vi "HFRR ADV v07.vi"() -> ()   [LabVIEW 2025] (continued)
                n2727 = local read "export"() -> (w3522:string)
                n2728 = call <vilib>:"Write Characters To File.vi"("append to file? (new file:F)"=FALSE, "character string"=w3522, "file path (dialog if empty)"=w3527) -> ()  [unwired: 2 in, 1 out]
              }
            }
          }
          frame Enabled {
          }
        }
        n2729 = case shown="True" "OK Button 17" {
          frame False {
          }
          frame True {
            (unwired) 0  # existing file
            w3780 = "Choose a datalog file to open"  # prompt
            n2730 = local write "OK Button 17"(FALSE ("OK Button 17")) -> ()
            n2731 = local read "String"() -> (w3775:string)
            n2732 = String To Path(string=w3775) -> (path=w3776:path)
            n2733 = File Dialog(6:"*.duf" ("pattern"), 7:w3780, 11:w3776) -> (0:w3767:errorcluster, 3:w3786:path)  [unwired: 4 in, 2 out]
            n2734 = Unbundle(w3767) -> ()  [unwired: 3 out]
            n2735 = Open/Create/Replace File "Open File"(file path (use dialog)=w3786) -> (refnum out=w3778:refnum<file>)  [unwired: 5 in, 2 out]
            n2736 = Strip Path(path=w3786) -> (name=w3784:string)  [unwired: 1 out]
            n2737 = Path To String(path=w3786) -> (string=w3769:string)
            n2738 = local write "String 29"(w3769) -> ()
            n2739 = while {
              tunnel: w3778 -> [w3790]
              i -> [w3787]
              stop <- w3788 continue-if-true
              (unwired) TRUE ("line mode (F)")
              n2740 = Read from Text File "Read File"(file (use dialog)=w3790) -> (text=w3789:string)  [unwired: 3 in, 3 out]
              n2741 = local write "Numeric 16"(w3787) -> ()
              n2742 = String Length(string=w3789) -> (length=w3792:i32)
              n2743 = Greater?(x=w3792, y=1) -> (0:w3788:bool)
            }
            n2744 = Search and Replace String(input string=w3769, search string=".duf", replace string=".dgf" ("replace string (\"\")")) -> (result string=→"String Indicator 4":string)  [unwired: 5 in, 3 out]
            n2745 = Match Pattern(string=w3784, regular expression=".dwm") -> (before substring=w3768:string)  [unwired: 1 in, 3 out]
            "String Indicator" <- w3768
            n2746 = Match Pattern(string=w3769, regular expression=".dwm" ("substring (\"\")")) -> (before substring=w3770:string)  [unwired: 1 in, 3 out]
            "String Indicator 3" <- w3770
            n2747 = local write "TITTLE 2"(w3768) -> ()
            n2748 = String To Path(string=w3770) -> (path=w3777:path)
            "path" <- w3777
            n2749 = call <vilib>:"Read Characters From File.vi"("file path (dialog if empty)"=w3777, "start of read offset (chars.:0)"=60 ("start of read offset (chars.: 0)")) -> ("character string"=→"String Indicator 2":string)  [unwired: 4 in, 3 out]
          }
        }
        n2750 = case shown="True" "Print 2" {
          frame False {
          }
          frame True {
            n2751 = flat-sequence {
              frame #0 {
                n2752 = local read "s.NO"() -> (→"s.NO 2":string)
                n2753 = Wait (ms)(milliseconds to wait=u32 20) -> ()  [unwired: 1 out]
                n2754 = local read "Sample ID  4"() -> (→"Sample ID  7":string)
                n2755 = local read "Sample ID  3"() -> (→"Sample ID  6":string)
                n2756 = local read "Sample ID"() -> (→"Sample ID  2":string)
                n2757 = local read "Tested by"() -> (→"Tested by 2":string)
                n2758 = local read "Test Date"() -> (→"Test Date 2":string)
                n2759 = local read "Humidity after test 3"() -> (→"Humidity after test 4":dbl)
                n2760 = local read "Ref A Test Date :"() -> (→"TITTLE 4":string)
                n2761 = local read "Temperature before test 3"() -> (→"Temperature after test 5":dbl)
                n2762 = local read "Temperature before test 3"() -> (w3588:dbl)
                n2763 = local read "Temperature after test 3"() -> (→"Temperature after test 4":dbl)
                n2764 = local read "Humidity before test 3"() -> (→"Humidity before test 4":dbl)
                n2765 = local write "Temperature before test 3"(w3588) -> ()
                n2766 = local read "image data"() -> (w3579:T13)
                n2767 = String To Path(string="C:\\LAB-IQ\\im\\Temp_resized.jpg") -> (path=w3580:path)
                "path 2" <- w3580
                n2768 = call <vilib>:"Write JPEG File.vi"("image data"=w3579, "path to JPEG file"=w3580) -> ()  [unwired: 8 in, 2 out]
                "Ref A Test Date :" <- "Ref A Test Date :"
                "Ref B Test Date :" <- "Ref B Test Date :"
                "Ref B Scar Value :" <- "Ref B Scar Value :"
                "Ref A Scar Value :" <- "Ref A Scar Value :"
              }
              frame #1 {
                (unwired) HTML_Report_Image_Alignment."MIDDLE" ("alignment (default)")
                w3616 = u16 0 items=["portrait", "landscape"] ("orientation (portrait)")
                (unwired) HTML_Report_Image_Alignment."ABSMIDDLE" ("alignment (default)")
                (unwired) "TESTED BY : "
                (unwired) "TESTED DATE :"
                (unwired) "SAMPLE ID : "
                (unwired) "SAMPLE DESIGN : "
                w3649 = "\r"
                # "add image"
                n2769 = Wait (ms)(milliseconds to wait=u32 20) -> ()  [unwired: 1 out]
                n2770 = local read "Sample ID  2"() -> (w3642:string)
                n2771 = local read "Wear Scar X"() -> (w3614:dbl)
                "Length ( microns ) 2" <- w3614
                n2772 = local read "Wear Scar Y"() -> (w3613:dbl)
                "Wear Scar Y ( microns ) :" <- w3613
                n2773 = local read "Test Date 2"() -> (w3643:string)
                n2774 = local read "Tested by 2"() -> (w3644:string)
                n2775 = local read "String 46"() -> (w3640:string)
                n2776 = local read "String 47"() -> (w3645:string)
                n2777 = local read "String 48"() -> (w3646:string)
                n2778 = local read "String 49"() -> (w3647:string)
                n2779 = local read "String 10"() -> (w3600:string)
                n2780 = local read "s.NO 2"() -> (w3641:string)
                n2781 = Add(x=w3614, y=w3613) -> (x+y=w3612:dbl)
                n2782 = call <vilib>:"New Report.vi"("report type"=enum16{"Standard Report", "HTML"}."HTML") -> ("report out"=w3620:refnum<class "NI_report.lvclass">, "error out"=w3618:errorcluster)  [unwired: 13 in]
                n2783 = Concatenate Strings(w3649, w3640, w3641, w3649, w3646, w3642, w3649, w3645, w3643, w3649, w3647, w3644, w3649) -> (→"test by 2":string)
                n2784 = Concatenate Strings("C:\\LAB-IQ\\Data\\" ("string"), w3600, ".jpg" ("string")) -> ()  [unwired: 1 out]
                n2785 = Divide(x=w3612, y=2.0) -> (x/y=→"Mean Wear ( microns) :":dbl)
                n2786 = call-dynamic "Set Report Orientation.vi"("report in"=w3620, "orientation (portrait)"=w3616, "error in (no error)"=w3618) -> ("report out"=w3619:refnum<class "NI_report.lvclass">, "error out"=w3617:errorcluster)  [unwired: 11 in]
                n2787 = for {
                  N: 5 -> [_]
                  tunnel: w3619 -> [w3670]
                  tunnel: [w3669] -> w3598
                  tunnel: w3617 -> [w3668]
                  tunnel: [w3667] -> w3597
                  n2788 = call-dynamic "Set Report Tab Width.vi"("report in"=w3670, "error in (no error)"=w3668) -> ("report out"=w3669:refnum<class "NI_report.lvclass">, "error out"=w3667:errorcluster)  [unwired: 12 in]
                }
                n2789 = local read "TITTLE"() -> (w3615:string)
                n2790 = call-dynamic "Set Report Header Text.vi"("report in"=w3598, "center header text"=w3615, "error in (no error)"=w3597) -> ("report out"=w3636:refnum<class "NI_report.lvclass">, "error out"=w3635:errorcluster)  [unwired: 11 in]
                n2791 = for {
                  N: 1 -> [_]
                  tunnel: [w3674] -> w3622
                  tunnel: [w3673] -> w3621
                  tunnel: w3636 -> [w3672]
                  tunnel: w3635 -> [w3671]
                  n2792 = call-dynamic "New Report Line.vi"("report in"=w3672, "error in (no error)"=w3671) -> ("report out"=w3674:refnum<class "NI_report.lvclass">, "error out"=w3673:errorcluster)  [unwired: 12 in]
                }
                n2793 = for {
                  N: 2 -> [_]
                  tunnel: [w3666] -> w3628
                  tunnel: [w3665] -> w3627
                  tunnel: w3622 -> [w3664]
                  tunnel: w3621 -> [w3663]
                  n2794 = call-dynamic "New Report Line.vi"("report in"=w3664, "error in (no error)"=w3663) -> ("report out"=w3666:refnum<class "NI_report.lvclass">, "error out"=w3665:errorcluster)  [unwired: 12 in]
                }
                n2795 = for {
                  N: 25 -> [_]
                  tunnel: w3628 -> [w3662]
                  tunnel: w3627 -> [w3660]
                  tunnel: [w3661] -> w3631
                  tunnel: [w3659] -> w3630
                  n2796 = call-dynamic "Set Report Tab Width.vi"("report in"=w3662, "error in (no error)"=w3660) -> ("report out"=w3661:refnum<class "NI_report.lvclass">, "error out"=w3659:errorcluster)  [unwired: 12 in]
                }
                n2797 = control-ref of="Tab Control 9"() -> (w3626:refnum<vi>)
                n2798 = call-dynamic "Append Control Image to Report.vi"("report in"=w3631, "alignment (default)"=HTML_Report_Image_Alignment."ABSMIDDLE", "ctrl reference"=w3626, "error in (no error)"=w3630) -> ("report out"=w3625:refnum<class "NI_report.lvclass">, "error out"=w3624:errorcluster)  [unwired: 8 in, 2 out]
                n2799 = for {
                  N: 3 -> [_]
                  tunnel: [w3658] -> w3609
                  tunnel: [w3657] -> w3608
                  tunnel: w3625 -> [w3656]
                  tunnel: w3624 -> [w3655]
                  n2800 = call-dynamic "New Report Line.vi"("report in"=w3656, "error in (no error)"=w3655) -> ("report out"=w3658:refnum<class "NI_report.lvclass">, "error out"=w3657:errorcluster)  [unwired: 12 in]
                }
                n2801 = for {
                  N: 100 -> [_]
                  tunnel: w3609 -> [w3654]
                  tunnel: w3608 -> [w3652]
                  tunnel: [w3653] -> w3605
                  tunnel: [w3651] -> w3603
                  n2802 = call-dynamic "Set Report Tab Width.vi"("report in"=w3654, "error in (no error)"=w3652) -> ("report out"=w3653:refnum<class "NI_report.lvclass">, "error out"=w3651:errorcluster)  [unwired: 12 in]
                }
                n2803 = String To Path(string="C:\\LAB-IQ\\im\\Temp_resized.jpg") -> (path=w3595:path)
                n2804 = call-poly <vilib>:"Append Image to Report.vi"("report in"=w3605, "path or URL of image"=w3595, "error in (no error)"=w3603) -> ("report out"=w3604:refnum<class "NI_report.lvclass">, "error out"=w3602:errorcluster)  [unwired: 9 in, 2 out]
                n2805 = call-poly <vilib>:"Open HTML Report in Browser.vi"("report in"=w3604, "error in (no error)"=w3602) -> ("report out"=w3639:refnum<class "NI_report.lvclass">, "error out"=w3638:errorcluster)  [unwired: 11 in, 1 out]
                n2806 = call-dynamic "Dispose Report.vi"("report in"=w3639, "error in (no error)"=w3638) -> ()  [unwired: 13 in, 1 out]
              }
              frame #2 {
              }
              frame #3 {
                n2807 = local write "Print 2"(FALSE ("Print")) -> ()
                n2808 = disable-structure shown="Disabled" {
                  frame Disabled {
                    n2809 = local read "String 10"() -> (w3679:string)
                    n2810 = Concatenate Strings("C:\\LAB-IQ-NXT\\Data\\" ("string"), w3679, ".jpg" ("string")) -> (w3677:string)
                    n2811 = String To Path(string=w3677) -> (path=w3676:path)
                    n2812 = Delete(path (use dialog)=w3676) -> ()  [unwired: 4 in, 3 out]
                  }
                  frame Enabled {
                  }
                }
              }
            }
          }
        }
        n2813 = case shown="True" w3466 {
          frame False {
          }
          frame True {
            n2814 = flat-sequence {
              frame #0 {
              }
              frame #1 {
                n2815 = Wait (ms)(milliseconds to wait=u32 100) -> ()  [unwired: 1 out]
              }
              frame #2 {
                n2816 = local write "OK Button 16"(FALSE ("Print 3")) -> ()
              }
            }
          }
        }
        n2817 = case shown="True" "Print" {
          tunnel: w3471 -> [_ w3763]
          frame False {
          }
          frame True {
            (unwired) i16 6 ("width (-)")
            (unwired) "TESTED BY : "
            (unwired) "TESTED DATE :"
            (unwired) "SAMPLE ID : "
            (unwired) "SAMPLE DESIGN : "
            w3721 = "\r"
            w3738 = "\r"
            # "add image"
            n2818 = local read "Sample ID"() -> (w3711:string)
            n2819 = local read "Tested by"() -> (w3714:string)
            n2820 = local read "String 45"() -> (w3681:string)
            n2821 = local read "Test Date"() -> (w3712:string)
            n2822 = local read "String 39"() -> (w3684:string)
            n2823 = local read "String 38"() -> (w3687:string)
            n2824 = local read "String 37"() -> (w3694:string)
            n2825 = local read "String 36"() -> (w3691:string)
            n2826 = local read "String 35"() -> (w3696:string)
            n2827 = local read "String 34"() -> (w3701:string)
            n2828 = local read "String 31"() -> (w3715:string)
            n2829 = local read "String 32"() -> (w3716:string)
            n2830 = local read "String 33"() -> (w3717:string)
            n2831 = local write "Print"(FALSE ("Print FF")) -> ()
            n2832 = local read "S 39"() -> (w3699:string)
            n2833 = local read "S 38"() -> (w3706:string)
            n2834 = local read "Temperature before test 2"() -> (w3737:dbl)
            n2835 = local read "Temperature after test 2"() -> (w3727:dbl)
            n2836 = local read "Humidity before test 2"() -> (w3752:dbl)
            n2837 = local read "Humidity after test 2"() -> (w3736:dbl)
            n2838 = local read "MWSD 2"() -> (w3741:dbl)
            n2839 = local read "WS1.4 2"() -> (w3719:dbl)
            n2840 = Concatenate Strings("8)" ("string"), w3684) -> (w3685:string)
            n2841 = Concatenate Strings("7)" ("string"), w3687) -> (w3688:string)
            n2842 = Concatenate Strings("6)" ("string"), w3691) -> (w3690:string)
            n2843 = Concatenate Strings("5)" ("string"), w3694) -> (w3693:string)
            n2844 = Concatenate Strings("4)" ("string"), w3696) -> (w3697:string)
            n2845 = Concatenate Strings("3)" ("string"), w3699) -> (w3700:string)
            n2846 = Concatenate Strings("2)" ("string"), w3701) -> (w3702:string)
            n2847 = Concatenate Strings("1)" ("string"), w3706) -> (w3705:string)
            n2848 = local read "HCF 2"() -> (w3723:dbl)
            n2849 = local read "AVP 2"() -> (w3740:dbl)
            n2850 = local read "s.NO"() -> (w3682:string)
            n2851 = call <vilib>:"New Report.vi"("report type"=enum16{"Standard Report", "HTML"}."Standard Report") -> ("report out"=w3761:refnum<class "NI_report.lvclass">, "error out"=w3760:errorcluster)  [unwired: 13 in]
            n2852 = local read "TITTLE"() -> (w3713:string)
            n2853 = Concatenate Strings(w3738, w3681, w3682, w3738, w3716, w3711, w3738, w3715, w3712, w3738, w3717, w3714, w3738) -> (w3731:string)
            "test by" <- w3731
            n2854 = Number To Fractional String(number=w3719, precision (6)=i16 2) -> (F-format string=w3718:string)  [unwired: 2 in]
            n2855 = Number To Fractional String(number=w3723, width (-)=i16 6, precision (6)=i16 2) -> (F-format string=w3722:string)  [unwired: 1 in]
            n2856 = Number To Fractional String(number=w3727, width (-)=i16 6, precision (6)=i16 2) -> (F-format string=w3728:string)  [unwired: 1 in]
            n2857 = Number To Fractional String(number=w3740, width (-)=i16 6, precision (6)=i16 2) -> (F-format string=w3742:string)  [unwired: 1 in]
            n2858 = Number To Fractional String(number=w3741, width (-)=i16 6, precision (6)=i16 2) -> (F-format string=w3743:string)  [unwired: 1 in]
            n2859 = Number To Fractional String(number=w3736, width (-)=i16 6, precision (6)=i16 2) -> (F-format string=w3739:string)  [unwired: 1 in]
            n2860 = Number To Fractional String(number=w3737, width (-)=i16 6, precision (6)=i16 2) -> (F-format string=w3726:string)  [unwired: 1 in]
            n2861 = Number To Fractional String(number=w3752, width (-)=i16 6, precision (6)=i16 2) -> (F-format string=w3757:string)  [unwired: 1 in]
            n2862 = call-dynamic "Set Report Header Text.vi"("report in"=w3761, "center header text"=w3713, "error in (no error)"=w3760) -> ("report out"=w3732:refnum<class "NI_report.lvclass">, "error out"=w3733:errorcluster)  [unwired: 11 in]
            n2863 = Concatenate Strings(w3721, w3705, w3757, w3721, w3702, w3726, w3721, w3700, w3739, w3721, w3697, w3728, w3721, w3693, w3743, w3721, w3690, w3742, w3721, w3688, w3722, w3721, w3685, w3718) -> (w3709:string)
            "export 2" <- w3709
            n2864 = call-poly <vilib>:"Append Report Text.vi"("report in"=w3732, "text"=w3731, "error in (no error)"=w3733) -> ("report out"=w3735:refnum<class "NI_report.lvclass">, "error out"=w3734:errorcluster)  [unwired: 9 in, 2 out]
            n2865 = local read "test by"() -> (w3708:string)
            n2866 = local read "TITTLE"() -> (w3710:string)
            n2867 = call-poly <vilib>:"Append Report Text.vi"("report in"=w3735, "error in (no error)"=w3734) -> ("report out"=w3756:refnum<class "NI_report.lvclass">, "error out"=w3754:errorcluster)  [unwired: 10 in, 2 out]
            n2868 = Concatenate Strings(w3710, w3709, w3708) -> (→"output":string)
            n2869 = call-poly <vilib>:"Append Report Text.vi"("report in"=w3756, "text"=w3709, "error in (no error)"=w3754) -> ("report out"=w3755:refnum<class "NI_report.lvclass">, "error out"=w3753:errorcluster)  [unwired: 9 in, 2 out]
            n2870 = call-dynamic "Print Report.vi"("report in"=w3755, "printer name (default)"=w3763, "error in (no error)"=w3753) -> ("report out"=w3765:refnum<class "NI_report.lvclass">, "error out"=w3766:errorcluster)  [unwired: 11 in]
            n2871 = call-dynamic "Dispose Report.vi"("report in"=w3765, "error in (no error)"=w3766) -> ()  [unwired: 13 in, 1 out]
          }
        }
      }
    }
    n2872 = case shown="True" "Prog Uno" {
      frame False {
      }
      frame True {
        n2873 = stacked-sequence {
          frame #0 {
            n2874 = Delete(path (use dialog)=path "C:/LAB-IQ-NXT/UNOCOMPILE.bat" ("working directory")) -> ()  [unwired: 4 in, 3 out]
          }
          frame #1 {
            n2875 = local read "Com Port 1"() -> (w2226:refnum<visa-resource-name>)
            n2876 = Concatenate Strings("cmd.exe /c \"mode " ("command line"), w2226, ":1200,n,8,1\"\n" ("command line")) -> (w2231:string)
            n2877 = Concatenate Strings(w2231, "CD\\\nCD WinDucom\navrdude -C avrdude.conf -v -patmega328p -carduino -P" ("command line"), w2226, " -b115200 -D -Uflash:w:UNO_V20.hex:i\n" ("command line"), "\r") -> (w2233:string)
            "STR" <- w2233
            n2878 = call <vilib>:"Write Characters To File.vi"("append to file? (new file:F)"=FALSE, "character string"=w2233, "file path (dialog if empty)"=path "C:/LAB-IQ/UNOCOMPILE.bat" ("working directory")) -> ()  [unwired: 2 in, 1 out]
          }
          frame #2 {
            n2879 = disable-structure shown="Disabled" {
              frame Disabled {
                w2237 = "cmd.exe  /c \"C:\\LAB-IQ-NXT\\UNOCOMPILE.bat\"" ("string")
                n2880 = local write "Prog Uno"(FALSE ("run minimized? (F)")) -> ()
                n2881 = call <vilib>:"System Exec.vi"("expected output size  (4096)"=u32 65535, "run minimized? (F)"=FALSE, "wait until completion? (T)"=TRUE ("run minimized? (F)"), "working directory"=path "C:/LAB-IQ-NXT", "standard input"=w2237, "command line"=w2237) -> ("error out"=w2236:errorcluster, "standard output"=→"String 42":string)  [unwired: 2 in, 2 out]
                "error out 3" <- w2236
                n2882 = flat-sequence {
                  tunnel: w2236 -> [_]
                  frame #0 {
                  }
                }
              }
              frame Enabled {
              }
            }
          }
        }
      }
    }
    n2883 = case shown="True" "Prog Due" {
      frame False {
      }
      frame True {
        n2884 = stacked-sequence {
          frame #0 {
            n2885 = Delete(path (use dialog)=path "C:/LAB-IQ/DUECOMPILE.bat" ("working directory")) -> ()  [unwired: 4 in, 3 out]
          }
          frame #1 {
            n2886 = disable-structure shown="Disabled" {
              frame Disabled {
                n2887 = local read "visa due"() -> (w2208:string)
                n2888 = Concatenate Strings("cmd.exe /c \"mode " ("command line"), w2208, ":1200,n,8,1\"\n" ("command line")) -> (w2213:string)
                n2889 = Concatenate Strings(w2213, "CD\\\nCD WinDucom\nTIMEOUT 1\n bossac.exe -i -d --port=" ("command line"), w2208, " -U false -e -w -v -b DUE.bin -R\n" ("command line"), "\r") -> (w2215:string)
                "concatenated string 2" <- w2215
                n2890 = call <vilib>:"Write Characters To File.vi"("append to file? (new file:F)"=FALSE, "character string"=w2215, "file path (dialog if empty)"=path "C:/LAB-IQ-NXT/DUECOMPILE.bat" ("working directory")) -> ()  [unwired: 2 in, 1 out]
              }
              frame Enabled {
              }
            }
          }
          frame #2 {
            # "C:\\LAB-IQ-NXT\\DUECOMPILE.bat"
            n2891 = local write "Prog Due"(FALSE ("Prog Due")) -> ()
            n2892 = disable-structure shown="Disabled" {
              frame Disabled {
                w2220 = "cmd.exe  /c \"C:\\LAB-IQ-NXT\\DUECOMPILE.bat\"" ("string")
                n2893 = call <vilib>:"System Exec.vi"("expected output size  (4096)"=u32 65535, "run minimized? (F)"=FALSE, "wait until completion? (T)"=TRUE ("run minimized? (F)"), "working directory"=path "C:/LAB-IQ-NXT", "standard input"=w2220, "command line"=w2220) -> ("error out"=w2219:errorcluster, "standard output"=→"String 44":string)  [unwired: 2 in, 2 out]
                "error out 4" <- w2219
                n2894 = flat-sequence {
                  tunnel: w2219 -> [_]
                  frame #0 {
                  }
                }
              }
              frame Enabled {
              }
            }
          }
        }
      }
    }
    n2895 = property on="SetTemp" class="DigNum (strict)"("Disabled"=w1630) -> ()  [unwired: 2 in, 2 out]
    n2896 = Multiply(x=w1620, y=w1622) -> (x*y=w1621:dbl)
    n2897 = local read "MWSD"() -> (w1619:dbl)
    n2898 = Add(x=w1621, y=w1619) -> (x+y=→"WS1.4":dbl)
    n2899 = Wait (ms)(milliseconds to wait=u32 50) -> ()  [unwired: 1 out]
    n2900 = Wait (ms)(milliseconds to wait=u32 50) -> ()  [unwired: 1 out]
    n2901 = local read "Quit"() -> (w1618:bool)
  }
  n2902 = while {
    tunnel: [w3838] -> w46
    shift-right: [w3831] -> _
    shift-left: 0.0 -> [w3834]
    shift-right: [w3830] -> _
    shift-left: 0.0 -> [w3833]
    shift-right: [w3829] -> _
    shift-left: 400.0 ("vc_cmd") -> [w3832]
    stop <- w3838 stop-if-true
    # "PID LOGIC"
    n2903 = local read "RUN"() -> (w3836:bool)
    n2904 = local read "Auto Start Test"() -> (w3835:bool)
    n2905 = local read "START TEMP"() -> (w3827:bool)
    n2906 = Or(x=w3836, y=w3835) -> (x .or. y?=w3837:bool)
    n2907 = And(x=w3837, y=w3827) -> (x .and. y?=w3828:bool)
    n2908 = case shown="True" w3828 {
      tunnel: [400.0 ("out_vc_cmd") w3858] -> w3829
      tunnel: [w3841 w3860] -> w3830
      tunnel: [w3841 w3859] -> w3831
      tunnel: w3834 -> [_ w3848]
      tunnel: w3833 -> [_ w3847]
      tunnel: w3832 -> [_ w3846]
      frame False {
        w3841 = 0.0 ("error_out")
      }
      frame True {
        n2909 = local read "measured_stroke"() -> (w3849:dbl)
        n2910 = local read "Set Strk"() -> (w3843:dbl)
        n2911 = Add(x=w3843, y="STROKE ADD") -> (x+y=w3844:dbl)
        n2912 = formula code="// Zero-Hardcode Explicit Positional-Form PID Engine\n// Inputs: target_stroke, measured_stroke, dt, prev_error, integral_accumulator_in, prev_vc_cmd\n//         kp, ki, kd, max_step_change, max_amplitude, min_amplitude, startup_cmd\n// Outputs: vc_cmd, error_out, out_error, integral_accumulator_out, out_vc_cmd\n\n// 1. Calculate Tracking Error\nfloat current_error = target_stroke - measured_stroke;\nerror_out = current_error;\n\n// 2. Compute Proportional Term\nfloat p_term = kp * current_error;\n\n// 3. Compute Derivative Term\nfloat d_term = 0.0;\nif (dt > 0.0) {\n    d_term = kd * ((current_error - prev_error) / dt);\n}\n\n// 4. Update and Accumulate Integral Term\nfloat current_integral = integral_accumulator_in + (current_error * dt);\nfloat i_term = ki * current_integral;\n\n// 5. Calculate Ideal Target Command\nfloat ideal_command = startup_cmd + p_term + i_term + d_term;\n\n// 6. Anti-Windup Protection (Back-calculation method)\nif (ideal_command > max_amplitude) {\n    float excess = ideal_command - max_amplitude;\n    if (ki > 0.0) {\n        current_integral -= excess / ki;\n    }\n    ideal_command = max_amplitude;\n} else if (ideal_command < min_amplitude) {\n    float excess = ideal_command - min_amplitude;\n    if (ki > 0.0) {\n        current_integral -= excess / ki;\n    }\n    ideal_command = min_amplitude;\n}\n\n// 7. Apply Loop Rate Limiting (Protects voice coil from large voltage steps)\nfloat raw_adjustment = ideal_command - prev_vc_cmd;\n\nif (raw_adjustment > max_step_change) {\n    raw_adjustment = max_step_change;\n} else if (raw_adjustment < -max_step_change) {\n    raw_adjustment = -max_step_change;\n}\n\nfloat next_vc_cmd = prev_vc_cmd + raw_adjustment;\n\n// Final Output Safety Safeguard Clamping\nif (next_vc_cmd > max_amplitude) {\n    next_vc_cmd = max_amplitude;\n} else if (next_vc_cmd < min_amplitude) {\n    next_vc_cmd = min_amplitude;\n}\n\n// 8. Map to Shift Registers for memory persistence\nvc_cmd = next_vc_cmd;\nout_error = current_error;                     \nintegral_accumulator_out = current_integral;  \nout_vc_cmd = next_vc_cmd;"("target_stroke"=w3844, "measured_stroke"=w3849, "dt"="dt", "integral_accumulator_in"=w3847, "prev_error"=w3848, "prev_vc_cmd"=w3846, "kp"="kp", "ki"="ki", "kd"="kd", "max_step_change"="max_step_change", "max_amplitude"="max_amplitude", "min_amplitude"="min_amplitude", "startup_cmd"="startup_cmd") -> ("vc_cmd"=w3864:dbl, "out_error"=w3859:dbl, "integral_accumulator_out"=w3860:dbl, "out_vc_cmd"=w3858:dbl)  [unwired: 1 out]
        "output Vpp" <- w3864
        n2913 = Number To Fractional String(number=w3864, precision (6)=i16 1) -> (F-format string=w3862:string)  [unwired: 2 in]
        n2914 = Concatenate Strings("DAC;" ("string"), w3862) -> (w3845:string)
        n2915 = local write "Command"(w3845) -> ()
        "prev_error" <- w3848
        "integral_accumulator_in" <- w3847
        "prev_vc_cmd" <- w3846
      }
    }
    n2916 = Wait (ms)(milliseconds to wait=u32 20) -> ()  [unwired: 1 out]
    n2917 = local read "Quit"() -> (w3838:bool)
  }
  n2918 = Or(x=w42, y=w41) -> (x .or. y?=w43:bool)
  n2919 = Or(x=w39, y=w43) -> (x .or. y?=w48:bool)
  n2920 = control-ref of="new picture"() -> ()  [unwired: 1 out]
  n2921 = Or(x=w54, y=w48) -> (x .or. y?=w45:bool)
  n2922 = Or(x=w45, y=w46) -> (x .or. y?=w40:bool)
  n2923 = while {
    tunnel: [w3865] -> w53
    i -> [w3872]
    stop <- w3865 stop-if-true
    n2924 = local read "Quit"() -> (w3865:bool)
    n2925 = Equal To 0?(x=w3872) -> (x = 0?=w3870:bool)
    n2926 = call "Elapsed Time3"("Time Target (s)"=45.0, "Auto Reset"=TRUE) -> ("Time has Elapsed"=w3869:bool)  [unwired: 10 in, 7 out]
    n2927 = Wait (ms)(milliseconds to wait=u32 50) -> ()  [unwired: 1 out]
    n2928 = Or(x=w3869, y=w3870) -> (x .or. y?=w3871:bool)
    n2929 = case shown="True" w3871 {
      frame False {
      }
      frame True {
        n2930 = call <vilib>:"System Exec.vi"("run minimized? (F)"=TRUE, "error in (no error)"="error in (no error)", "command line"="powercfg.exe -change -monitor-timeout-ac 0") -> ("error out"=w3883:errorcluster)  [unwired: 5 in, 3 out]
        n2931 = call <vilib>:"System Exec.vi"("run minimized? (F)"=TRUE, "error in (no error)"=w3883, "command line"="powercfg.exe -change -disk-timeout-ac 0") -> ("error out"=w3882:errorcluster)  [unwired: 5 in, 3 out]
        n2932 = call <vilib>:"System Exec.vi"("run minimized? (F)"=TRUE, "error in (no error)"=w3882, "command line"="powercfg.exe -change -standby-timeout-ac 0") -> ("error out"=w3881:errorcluster)  [unwired: 5 in, 3 out]
        n2933 = call <vilib>:"System Exec.vi"("run minimized? (F)"=TRUE, "error in (no error)"=w3881, "command line"="powercfg.exe -change -hibernate-timeout-ac 0") -> ("error out"=w3880:errorcluster)  [unwired: 5 in, 3 out]
        n2934 = call <vilib>:"Simple Error Handler.vi"("error in (no error)"=w3880) -> ("error out"=w3886:errorcluster)  [unwired: 4 in, 4 out]
        n2935 = call <vilib>:"Clear Errors.vi"("error in (no error)"=w3886) -> ("error out"=→"error out":errorcluster)  [unwired: 5 in, 1 out]
      }
    }
  }
  n2936 = Compound Arithmetic op=OR(w56, w40, w53) -> (w55:bool)
  n2937 = flat-sequence {
    tunnel: w55 -> [_]
    tunnel: [w3888] -> w18
    tunnel: w18 -> [_]
    frame #0 {
      n2938 = call "CLOSE CONNECTION.vi"() -> ("error out"=w3888:errorcluster)  [unwired: 11 in]
    }
    frame #1 {
      n2939 = Quit LabVIEW(quit? (T)=TRUE) -> ()
      n2940 = local write "Quit"(FALSE ("EXIT")) -> ()
    }
  }
  n2941 = property on="Heater Button" class="Bool (strict)"("Visible"=TRUE) -> ()  [unwired: 2 in, 2 out]
  n2942 = disable-structure shown="Disabled" {
    disable-tunnel: _ -> [w3894 _]
    disable-tunnel: _ -> [w3891 _]
    disable-tunnel: _ -> [w3892 _]
    frame Disabled {
      n2943 = disable-structure shown="Disabled" {
        disable-tunnel: [w3901 _] -> w3893
        frame Disabled {
          n2944 = while {
            shift-right: [w3943] -> w3899
            shift-left: errorcluster {"status"=TRUE, "code"=0, "source"="Init"} ("error out") -> [w3908]
            shift-right: [w3942] -> w3898
            shift-left: _ -> [w3909]
            shift-right: [w3941] -> _
            shift-left: "" -> [w3940]
            tunnel: [w3902] -> w3901
            shift-right: ["Set Rh"] -> _
            shift-left: 0.0 ("Set Rh") -> [w3934]
            tunnel: [w3911] -> _
            i -> [w3911]
            stop <- w3902 stop-if-true
            n2945 = flat-sequence {
              tunnel: w3908 -> [w3946]
              tunnel: [w3946] -> w3907
              frame #0 {
                n2946 = Wait (ms)(milliseconds to wait=u32 200) -> ()  [unwired: 1 out]
              }
            }
            n2947 = local read "Com Port 3"() -> (w3910:refnum<visa-resource-name>)
            n2948 = local read "Humidity Str Rec"() -> (w3912:string)
            n2949 = Not Equal?(x="Set Rh", y=w3934) -> (x != y?=w3939:bool)
            n2950 = Number To Decimal String(number="Set Rh") -> (decimal integer string=w3937:string)  [unwired: 1 in]
            n2951 = Not Equal?(x=w3910, y=w3909) -> (x != y?=w3905:bool)
            n2952 = Concatenate Strings("#setPoint00" ("string"), w3937) -> (w3938:string)
            n2953 = case shown="False" w3939 {
              tunnel: w3938 -> [_ w3958]
              frame False {
                n2954 = local read "Humidity"() -> (w3955:bool)
                n2955 = case shown="True" w3955 {
                  frame False {
                    n2956 = local write "Humidity Str Send"("stop" ("Humidity Str Send")) -> ()
                  }
                  frame True {
                    n2957 = local write "Humidity Str Send"("start" ("Humidity Str Send")) -> ()
                  }
                }
              }
              frame True {
                n2958 = local write "Humidity Str Send"(w3958) -> ()
              }
            }
            n2959 = Or(x=w3905) -> (y=w3903:bool, x .or. y?=w3904:bool)
            n2960 = String Subset(string=w3912, offset (0)=7) -> (substring=w3927:string)  [unwired: 1 in]
            n2961 = Match Pattern(string=w3912, regular expression="?") -> (offset past match=w3930:i32)  [unwired: 1 in, 3 out]
            n2962 = Match Pattern(string=w3912, regular expression="v") -> (offset past match=w3933:i32)  [unwired: 1 in, 3 out]
            n2963 = case shown="True" w3904 {
              tunnel: w3907 -> [w3944 _]
              tunnel: [w3944 errorcluster {"status"=TRUE, "code"=0, "source"="Init"} ("error out")] -> w3906
              frame False {
              }
              frame True {
              }
            }
            n2964 = Equal?(x=w3930, y=-1) -> (x = y?=w3914:bool)
            n2965 = Match Pattern(string=w3927, regular expression="g") -> (after substring=w3928:string, offset past match=w3919:i32)  [unwired: 1 in, 2 out]
            n2966 = Match Pattern(string=w3927, regular expression="y") -> (after substring=w3926:string, offset past match=w3920:i32)  [unwired: 1 in, 2 out]
            n2967 = Greater?(x=w3920, y=w3919) -> (0:w3925:bool)
            n2968 = Greater Or Equal To 0?(x=w3920) -> (x >= 0?=w3917:bool)
            n2969 = Greater Or Equal To 0?(x=w3919) -> (x >= 0?=w3918:bool)
            n2970 = Or(x=w3917, y=w3918) -> (x .or. y?=w3916:bool)
            n2971 = Greater Or Equal To 0?(x=w3933) -> (x >= 0?=w3915:bool)
            n2972 = Select(t=w3926, s=w3925, f=w3928) -> (s? t:f=w3921:string)
            n2973 = case shown="Error" w3906 {
              selector: w3906 -> [w3971 w4017]
              tunnel: [w3969 w4010] -> w3943
              tunnel: w3909 -> [w3972 w4016]
              tunnel: [w3970 w4019] -> w3942
              tunnel: w3940 -> [w3959 w4018]
              tunnel: [w3966 w4018] -> w3941
              frame No Error {
                n2974 = call "Elapsed Time7"() -> ("Time has Elapsed"=w3965:bool)  [unwired: 12 in, 7 out]
                n2975 = Not Equal?(x="Humidity Str Send", y=w3959) -> (x != y?=w3961:bool)
                n2976 = Or(x=w3961, y=w3965) -> (x .or. y?=w3964:bool)
                n2977 = Select(t="Humidity Str Send", s=w3961, f="vals" ("regular expression")) -> (s? t:f=w3960:string)
                n2978 = Or(x=w3964, y="Send") -> (x .or. y?=w3968:bool)
                n2979 = case shown="True" w3968 {
                  tunnel: [w3975 w3980] -> w3969
                  tunnel: w3972 -> [w3974 w3988]
                  tunnel: w3971 -> [w3975 w3987]
                  tunnel: [w3974 w3981] -> w3970
                  tunnel: w3960 -> [_ w3986]
                  tunnel: [w3973 w3977] -> w3966
                  tunnel: "Humidity Str Send" -> [_ w3978]
                  tunnel: w3961 -> [_ w3979]
                  tunnel: w3959 -> [w3973 w3976]
                  frame False {
                  }
                  frame True {
                    n2980 = flat-sequence {
                      tunnel: w3988 -> [w3996]
                      tunnel: w3987 -> [w3995]
                      tunnel: w3986 -> [w3992]
                      tunnel: [w3994] -> w3985
                      tunnel: [w3993] -> w3984
                      tunnel: w3985 -> [w3999]
                      tunnel: w3984 -> [w3998]
                      tunnel: [w3999] -> w3983
                      tunnel: [w3998] -> w3982
                      tunnel: w3983 -> [w4006]
                      tunnel: w3982 -> [w4005]
                      tunnel: [w4004] -> w3981
                      tunnel: [w4003] -> w3980
                      frame #0 {
                        n2981 = local write "Ser Led"(TRUE ("Boolean 4")) -> ()
                        n2982 = Concatenate Strings(w3992, "\r") -> (w3991:string)
                        n2983 = VISA Write(VISA resource name=w3996, write buffer=w3991, error in (no error)=w3995) -> (VISA resource name out=w3994:refnum<visa-resource-name>, error out=w3993:errorcluster)  [unwired: 1 out]
                      }
                      frame #1 {
                        n2984 = Wait (ms)(milliseconds to wait="wait") -> ()  [unwired: 1 out]
                      }
                      frame #2 {
                        w4001 = FALSE ("Send")
                        n2985 = property class="Instr"(reference=w4006, error in=w4005) -> (reference out=w4007:refnum<visa-resource-name>, error out=w4008:errorcluster, "Serial Settings:Number of Bytes at Serial Port"=w4000:u32)
                        n2986 = local write "Send"(w4001) -> ()
                        n2987 = local write "Ser Led"(w4001) -> ()
                        n2988 = VISA Read(VISA resource name=w4007, byte count=w4000, error in (no error)=w4008) -> (VISA resource name out=w4004:refnum<visa-resource-name>, read buffer=→"Humidity Str Rec":string, error out=w4003:errorcluster)  [unwired: 1 out]
                      }
                    }
                    n2989 = Select(t=w3978, s=w3979, f=w3976) -> (s? t:f=w3977:string)
                  }
                }
              }
              frame Error {
                w4024 = u16 0 items=["None"=0, "XON/XOFF"=1, "RTS/CTS"=2, "DTR/DSR"=4] ("flow control")
                w4020 = u16 0 items=["None", "Odd", "Even", "Mark", "Space"] ("parity")
                w4023 = u16 10 items=["1.0"=10, "1.5"=15, "2.0"=20] ("stop bits")
                n2990 = VISA Close(VISA resource name=w4016, error in (no error)=w4017) -> (error out=w4015:errorcluster)
                n2991 = local write "humid"("" ("humid")) -> ()
                n2992 = local write "Humidity Str Rec"("" ("Humidity Str Rec")) -> ()
                n2993 = call <vilib>:"Clear Errors.vi"("error in (no error)"=w4015) -> ("error out"=w4014:errorcluster)  [unwired: 5 in, 1 out]
                n2994 = local read "Com Port 3"() -> (w4013:refnum<visa-resource-name>)
                n2995 = call-poly "VISA Configure Serial Port"("VISA resource name"=w4013, "timeout (10sec)"=u32 1000, "termination char\n(0xA = '\\n' = LF)"=u8 10 ("termination char\n(0xA = '\\n' = LF)"), "Enable Termination\nChar (T)"=FALSE ("Enable Termination Char (T)"), "data bits (8)"=u16 8 ("data bits"), "parity (0:none)"=w4020, "error in (no error)"=w4014, "stop bits (10: 1 bit)"=w4023, "flow control (0:none)"=w4024) -> ("VISA resource name out"=w4019:refnum<visa-resource-name>, "baud rate (9600)"=w4011:u32, "error out"=w4010:errorcluster)  [unwired: 4 in]
              }
            }
            n2996 = Compound Arithmetic op=AND(w3915, w3914, w3916) -> (w3913:bool)
            n2997 = case shown="True" w3913 {
              tunnel: w3912 -> [_ _]
              tunnel: w3921 -> [_ w3951]
              frame False {
              }
              frame True {
                w3949 = " " ("regular expression")
                n2998 = Match Pattern(string=w3951, regular expression=" ") -> (after substring=w3953:string)  [unwired: 1 in, 3 out]
                n2999 = Match Pattern(string=w3953, regular expression=w3949) -> (before substring=→"humid":string, after substring=w3950:string)  [unwired: 1 in, 2 out]
                n3000 = Match Pattern(string=w3950, regular expression=w3949) -> (before substring=→"temp_@Rh sensor":string)  [unwired: 1 in, 3 out]
              }
            }
            n3001 = local read "Quit"() -> (w3902:bool)
          }
          n3002 = VISA Close(VISA resource name=w3898, error in (no error)=w3899) -> (error out=w3895:errorcluster)
          n3003 = call <vilib>:"Clear Errors.vi"("error in (no error)"=w3895) -> ()  [unwired: 5 in, 2 out]
        }
        frame Enabled {
        }
      }
    }
    frame Enabled {
    }
  }
  n3004 = while {
    tunnel: [w4031] -> _
    i -> [w4031]
    stop <- w4027 stop-if-true
    # "Langauage selection"
    n3005 = Equal?(x="Lan flag", y=22.0) -> ()  [unwired: 1 out]
    n3006 = disable-structure shown="Disabled" {
      frame Disabled {
        n3007 = stacked-sequence {
          frame #0 {
            n3008 = case shown="\"Russian\"" "Language Selection" {
              tunnel: [0 1] -> w4033
              frame "English", Default {
              }
              frame "Russian" {
              }
            }
            n3009 = for {
              N: 130 -> [_]
              tunnel: "Table" -> [w4042]
              tunnel: w4033 -> [w4041]
              i -> [w4040]
              n3010 = Index Array(array=w4042, index (row)=w4040, index (col)=w4041) -> (element=w4039:string)
              n3011 = case shown="123" w4040 {
                tunnel: w4039 -> [w4043 w4044 _ w4045 w4046 w4047 w4048 w4049 w4050 w4051 w4052 w4053 w4054 w4055 w4056 w4057 w4058 w4059 w4060 w4061 w4062 w4063 w4064 w4065 w4066 w4067 w4068 w4069 w4070 _ _ w4071 w4072 w4073 w4074 w4075 w4076 w4085 w4092 w4099 w4106 w4110 w4113 w4116 w4118 w4120 w4121 w4122 w4123 w4124 w4125 w4126 w4127 w4128 w4129 w4130 w4131 w4132 w4133 w4134 w4135 w4136 w4137 w4138 w4139 w4140 w4141 w4142 w4143 w4144 w4145 w4146 w4147 w4148 w4149 w4150 w4151 w4152 w4153 w4154 w4155 w4156 w4157 w4158 w4159 w4160 w4161 w4162 w4163 w4164 w4165 w4166 w4167 w4168 w4169 w4170 w4171 w4172 w4173 w4174 w4175 w4176 w4177 w4178 w4179 _ w4180 w4181 w4182 w4183 w4184 w4185 w4186 w4187 w4188 w4189 w4190 w4191 w4192 _ w4193 w4194 w4195 w4196 w4197 w4198 _]
                frame 0 {
                  n3012 = local write "S"(w4043) -> ()
                }
                frame 1 {
                  n3013 = local write "S 2"(w4044) -> ()
                }
                frame 2 {
                }
                frame 3 {
                  n3014 = local write "S 4"(w4045) -> ()
                }
                frame 4 {
                  n3015 = property on="FILE" class="Str"("Caption.Text"=w4046) -> ()  [unwired: 2 in, 2 out]
                }
                frame 5 {
                  n3016 = property on="Fuel Discription :" class="Str"("Caption.Text"=w4047) -> ()  [unwired: 2 in, 2 out]
                }
                frame 6 {
                  n3017 = property on="Remarks :" class="Str"("Caption.Text"=w4048) -> ()  [unwired: 2 in, 2 out]
                }
                frame 7 {
                  n3018 = property on="Save & Continue" class="Bool (strict)"("Boolean Text.Text"=w4049) -> ()  [unwired: 2 in, 2 out]
                }
                frame 8 {
                }
                frame 9 {
                  n3019 = property on="Set Hz" class="DigNum (strict)"("Caption.Text"=w4051) -> ()  [unwired: 2 in, 2 out]
                }
                frame 10 {
                  "String 3" <- w4052
                }
                frame 11 {
                  n3020 = property on="NORMAL LOAD" class="DigNum (strict)"("Caption.Text"=w4053) -> ()  [unwired: 2 in, 2 out]
                }
                frame 12 {
                  "String 5" <- w4054
                }
                frame 13 {
                  n3021 = property on="Set Temp" class="DigNum (strict)"("Caption.Text"=w4055) -> ()  [unwired: 2 in, 2 out]
                }
                frame 14 {
                  n3022 = local write "S 15"(w4056) -> ()
                }
                frame 15 {
                  n3023 = property on="Set Rh" class="DigNum (strict)"("Caption.Text"=w4057) -> ()  [unwired: 2 in, 2 out]
                }
                frame 16 {
                  "String 13" <- w4058
                  "String 26" <- w4058
                }
                frame 17 {
                  n3024 = local write "S 18"(w4059) -> ()
                }
                frame 18 {
                  "String 17" <- w4060
                }
                frame 19 {
                  n3025 = property on="test time" class="DigNum (strict)"("Caption.Text"=w4061) -> ()  [unwired: 2 in, 2 out]
                }
                frame 20 {
                  "String 18" <- w4062
                  "String 22" <- w4062
                }
                frame 21 {
                  n3026 = property on="Elapsed time" class="DigNum (strict)"("Caption.Text"=w4063) -> ()  [unwired: 2 in, 2 out]
                }
                frame 22 {
                  n3027 = property on="Samplingtime 2" class="DigNum (strict)"("Caption.Text"=w4064) -> ()  [unwired: 2 in, 2 out]
                }
                frame 23 {
                  "String 21" <- w4065
                }
                frame 24 {
                  n3028 = property on="Countdown" class="DigNum (strict)"("Caption.Text"=w4066) -> ()  [unwired: 2 in, 2 out]
                }
                frame 25 {
                  n3029 = property on="Countdown 2" class="DigNum (strict)"("Caption.Text"=w4067) -> ()  [unwired: 2 in, 2 out]
                }
                frame 26 {
                  n3030 = property on="Engage" class="Bool (strict)"("Boolean Text.Text"=w4068) -> ()  [unwired: 2 in, 2 out]
                }
                frame 27 {
                  n3031 = property on="Boolean  4" class="Bool (strict)"("Boolean Text.Text"=w4069) -> ()  [unwired: 2 in, 2 out]
                }
                frame 28 {
                  n3032 = property on="Test \nStatus" class="Bool (strict)"("Boolean Text.Text"=w4070) -> ()  [unwired: 2 in, 2 out]
                }
                frame 29 {
                }
                frame 30 {
                }
                frame 31 {
                }
                frame 32 {
                  n3033 = property on="RSTCOF" class="Bool"("Boolean Text.Text"=w4072) -> ()  [unwired: 2 in, 2 out]
                  n3034 = property on="RST FF" class="Bool"("Boolean Text.Text"=w4072) -> ()  [unwired: 2 in, 2 out]
                  n3035 = property on="RST TEMP" class="Bool"("Boolean Text.Text"=w4072) -> ()  [unwired: 2 in, 2 out]
                  n3036 = property on="RSTV1 3" class="Bool"("Boolean Text.Text"=w4072) -> ()  [unwired: 2 in, 2 out]
                  n3037 = property on="rstv2" class="Bool"("Boolean Text.Text"=w4072) -> ()  [unwired: 2 in, 2 out]
                  n3038 = property on="RSTV1 2" class="Bool"("Boolean Text.Text"=w4072) -> ()  [unwired: 2 in, 2 out]
                  n3039 = property on="RST CP" class="Bool"("Boolean Text.Text"=w4072) -> ()  [unwired: 2 in, 2 out]
                }
                frame 33 {
                  "S 61" <- w4073
                }
                frame 34 {
                  "String 23" <- w4074
                }
                frame 35 {
                  n3040 = property on="Rh Before" class="DigNum (strict)"("Caption.Text"=w4075) -> ()  [unwired: 2 in, 2 out]
                }
                frame 36 {
                  n3041 = Match Pattern(string=w4076, regular expression=",") -> (before substring=→"bs":string, after substring=→"as":string)  [unwired: 1 in, 2 out]
                  n3042 = property on="Rh After" class="DigNum (strict)"("Caption.Text"=w4076) -> ()  [unwired: 2 in, 2 out]
                }
                frame 37 {
                  n3043 = Match Pattern(string=w4085, regular expression=",") -> (before substring=w4084:string, after substring=w4083:string)  [unwired: 1 in, 2 out]
                  "bs" <- w4084
                  "as" <- w4083
                  n3044 = Concatenate Strings(w4084, w4083) -> (w4080:string)
                  n3045 = property on="Humidity before test 2" class="DigNum (strict)"("Caption.Text"=w4080) -> ()  [unwired: 2 in, 2 out]
                  n3046 = property on="Humidity before test" class="DigNum (strict)"("Caption.Text"=w4080) -> ()  [unwired: 2 in, 2 out]
                  n3047 = Concatenate Strings(w4080, "=" ("string")) -> (w4081:string)
                  n3048 = local write "S 38"(w4081) -> ()
                }
                frame 38 {
                  n3049 = Match Pattern(string=w4092, regular expression=",") -> (before substring=w4091:string, after substring=w4090:string)  [unwired: 1 in, 2 out]
                  "bs" <- w4091
                  "as" <- w4090
                  n3050 = Concatenate Strings(w4091, w4090) -> (w4087:string)
                  n3051 = property on="Humidity after test 2" class="DigNum (strict)"("Caption.Text"=w4087) -> ()  [unwired: 2 in, 2 out]
                  n3052 = Concatenate Strings(w4087, "=" ("string")) -> (w4089:string)
                  n3053 = property on="Humidity after test" class="DigNum (strict)"("Caption.Text"=w4087) -> ()  [unwired: 2 in, 2 out]
                  n3054 = local write "S 39"(w4089) -> ()
                }
                frame 39 {
                  n3055 = Match Pattern(string=w4099, regular expression=",") -> (before substring=w4098:string, after substring=w4097:string)  [unwired: 1 in, 2 out]
                  "bs" <- w4098
                  "as" <- w4097
                  n3056 = Concatenate Strings(w4098, w4097) -> (w4094:string)
                  n3057 = property on="Temperature before test 2" class="DigNum (strict)"("Caption.Text"=w4094) -> ()  [unwired: 2 in, 2 out]
                  n3058 = property on="Temperature before test" class="DigNum (strict)"("Caption.Text"=w4094) -> ()  [unwired: 2 in, 2 out]
                  n3059 = Concatenate Strings(w4094, "=" ("string")) -> (→"String 34":string)
                }
                frame 40 {
                  n3060 = Match Pattern(string=w4106, regular expression=",") -> (before substring=w4105:string, after substring=w4104:string)  [unwired: 1 in, 2 out]
                  "bs" <- w4105
                  "as" <- w4104
                  n3061 = Concatenate Strings(w4105, w4104) -> (w4101:string)
                  n3062 = property on="Temperature after test 2" class="DigNum (strict)"("Caption.Text"=w4101) -> ()  [unwired: 2 in, 2 out]
                  n3063 = Concatenate Strings(w4101, "=" ("string")) -> (→"String 35":string)
                  n3064 = property on="Temperature after test" class="DigNum (strict)"("Caption.Text"=w4101) -> ()  [unwired: 2 in, 2 out]
                }
                frame 41 {
                  n3065 = property on="AVP" class="DigNum (strict)"("Caption.Text"=w4110) -> ()  [unwired: 2 in, 2 out]
                  n3066 = property on="AVP 2" class="DigNum (strict)"("Caption.Text"=w4110) -> ()  [unwired: 2 in, 2 out]
                  n3067 = Concatenate Strings(w4110, "=" ("string")) -> (→"String 36":string)
                }
                frame 42 {
                  n3068 = property on="MWSD" class="DigNum (strict)"("Caption.Text"=w4113) -> ()  [unwired: 2 in, 2 out]
                  n3069 = property on="MWSD 2" class="DigNum (strict)"("Caption.Text"=w4113) -> ()  [unwired: 2 in, 2 out]
                  n3070 = Concatenate Strings(w4113, "=" ("string")) -> (→"String 37":string)
                }
                frame 43 {
                  n3071 = property on="HCF 2" class="DigNum (strict)"("Caption.Text"=w4116) -> ()  [unwired: 2 in, 2 out]
                  n3072 = property on="HCF" class="DigNum (strict)"("Caption.Text"=w4116) -> ()  [unwired: 2 in, 2 out]
                  n3073 = Concatenate Strings(w4116, "=" ("string")) -> (→"String 38":string)
                }
                frame 44 {
                  n3074 = Concatenate Strings(w4118, "=" ("string")) -> (→"String 39":string)
                  n3075 = property on="WS1.4 2" class="DigNum (strict)"("Caption.Text"=w4118) -> ()  [unwired: 2 in, 2 out]
                  n3076 = property on="WS1.4" class="DigNum (strict)"("Caption.Text"=w4118) -> ()  [unwired: 2 in, 2 out]
                }
                frame 45 {
                  n3077 = property on="Save Results" class="Bool (strict)"("Boolean Text.Text"=w4120) -> ()  [unwired: 2 in, 2 out]
                }
                frame 46 {
                  n3078 = local write "S 47"(w4121) -> ()
                }
                frame 47 {
                  n3079 = local write "S 48"(w4122) -> ()
                }
                frame 48 {
                  n3080 = local write "S 49"(w4123) -> ()
                }
                frame 49 {
                  n3081 = local write "S 50"(w4124) -> ()
                }
                frame 50 {
                  n3082 = local write "S 51"(w4125) -> ()
                }
                frame 51 {
                  n3083 = local write "S 52"(w4126) -> ()
                }
                frame 52 {
                  n3084 = local write "S 53"(w4127) -> ()
                }
                frame 53 {
                  n3085 = local write "S 54"(w4128) -> ()
                }
                frame 54 {
                  n3086 = local write "S 55"(w4129) -> ()
                }
                frame 55 {
                  n3087 = local write "S 56"(w4130) -> ()
                }
                frame 56 {
                  n3088 = local write "S 57"(w4131) -> ()
                }
                frame 57 {
                  n3089 = local write "S 58"(w4132) -> ()
                }
                frame 58 {
                  n3090 = local write "S 59"(w4133) -> ()
                }
                frame 59 {
                  n3091 = local write "S 60"(w4134) -> ()
                }
                frame 60 {
                  n3092 = local write "S 62"(w4135) -> ()
                }
                frame 61 {
                  n3093 = local write "S 63"(w4136) -> ()
                }
                frame 62 {
                  n3094 = local write "S 64"(w4137) -> ()
                }
                frame 63 {
                  n3095 = local write "S 65"(w4138) -> ()
                }
                frame 64 {
                  n3096 = local write "S 66"(w4139) -> ()
                }
                frame 65 {
                  n3097 = local write "S 67"(w4140) -> ()
                }
                frame 66 {
                  n3098 = local write "S 68"(w4141) -> ()
                }
                frame 67 {
                  n3099 = local write "S 69"(w4142) -> ()
                }
                frame 68 {
                  n3100 = local write "S 70"(w4143) -> ()
                }
                frame 69 {
                  n3101 = local write "S 71"(w4144) -> ()
                }
                frame 70 {
                  n3102 = local write "S 72"(w4145) -> ()
                }
                frame 71 {
                  n3103 = local write "S 73"(w4146) -> ()
                }
                frame 72 {
                  n3104 = local write "S 74"(w4147) -> ()
                }
                frame 73 {
                  n3105 = local write "S 75"(w4148) -> ()
                }
                frame 74 {
                  n3106 = local write "S 76"(w4149) -> ()
                }
                frame 75 {
                  n3107 = local write "S 77"(w4150) -> ()
                }
                frame 76 {
                  n3108 = local write "S 78"(w4151) -> ()
                }
                frame 77 {
                  n3109 = local write "S 79"(w4152) -> ()
                }
                frame 79 {
                  n3110 = property on="Sample Temperature ( °C )" class="XYGraph (strict)"("Y Scale.Name Label.Text"=w4153) -> ()  [unwired: 2 in, 2 out]
                }
                frame 80 {
                  n3111 = local write "S 81"(w4154) -> ()
                  n3112 = property on="Humidity ( %RH )" class="XYGraph (strict)"("Y Scale.Name Label.Text"=w4154) -> ()  [unwired: 2 in, 2 out]
                }
                frame 78 {
                  n3113 = property on="Air Temperature  ( °C )" class="XYGraph (strict)"("X Scale.Name Label.Text"=w4155) -> ()  [unwired: 2 in, 2 out]
                  n3114 = property on="Humidity ( %RH )" class="XYGraph (strict)"("X Scale.Name Label.Text"=w4155) -> ()  [unwired: 2 in, 2 out]
                  n3115 = property on="Sample Temperature ( °C )" class="XYGraph (strict)"("X Scale.Name Label.Text"=w4155) -> ()  [unwired: 2 in, 2 out]
                  n3116 = property on="Coefficient Of Friction" class="XYGraph (strict)"("X Scale.Name Label.Text"=w4155) -> ()  [unwired: 2 in, 2 out]
                }
